vi "Get Value (Numeric).vi"(8 "error in (no error)":errorcluster, 10 "key":string, 11 "JSON Object in":refnum<class "JSON Object.lvclass">) -> (0 "error out":errorcluster, 1 "found":bool, 2 "value":refnum<class "JSON Numeric.lvclass">)   [LabVIEW 2015, in "LVJSON.lvlib" / "JSON Object.lvclass"]
uses:
  JSON Object.lvclass
  JSON Numeric/JSON Numeric.lvclass
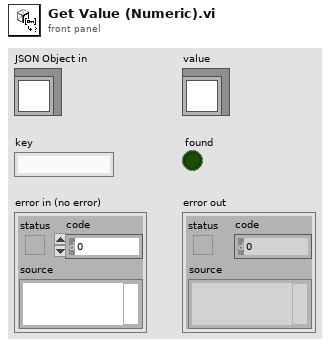
[diagram p1: front panel]
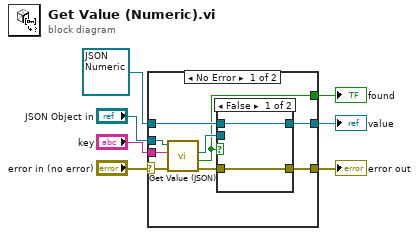
[diagram p0: block diagram]
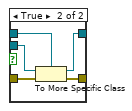
[diagram p2: hidden frame]
diagram:
  n1 = case shown="No Error" "error in (no error)" {
    selector: "error in (no error)" -> [w14 w25]
    tunnel: [w10 w25] -> w6
    tunnel: "JSON Object in" -> [w16 _]
    tunnel: "key" -> [w15 _]
    tunnel: [w12 w24] -> w2
    tunnel: refnum<class "JSON Numeric.lvclass"> refnum ("JSON Numeric.lvclass") -> [w9 w24]
    tunnel: [w8 _] -> w1
    frame No Error {
      n2 = call "Get Value (JSON).vi"("error in (no error)"=w14, "key"=w15, "JSON Object in"=w16) -> ("error out"=w11:errorcluster, "found"=w8:bool, "value"=w13:refnum<class "JSON Datatype.lvclass">)  [unwired: 6 in]
      n3 = case shown="False" w8 {
        tunnel: w13 -> [_ w23]
        tunnel: [w18 w22] -> w12
        tunnel: w11 -> [w17 w21]
        tunnel: [w17 w20] -> w10
        tunnel: w9 -> [w18 w19]
        frame False {
        }
        frame True {
          n4 = To More Specific Class(target class=w19, reference=w23, error in=w21) -> (specific class reference=w22:refnum<class "JSON Numeric.lvclass">, error out=w20:errorcluster)
        }
      }
    }
    frame Error {
    }
  }
  "error out" <- w6
  "value" <- w2
  "found" <- w1
